vi "tdms读取.vi"() -> ()   [LabVIEW 2018]
panel:
  out "XY图":cluster{"Y":dbl[], "Y":dbl[]}[](graph)
  out "数据":waveform(dbl)[](array[waveform])
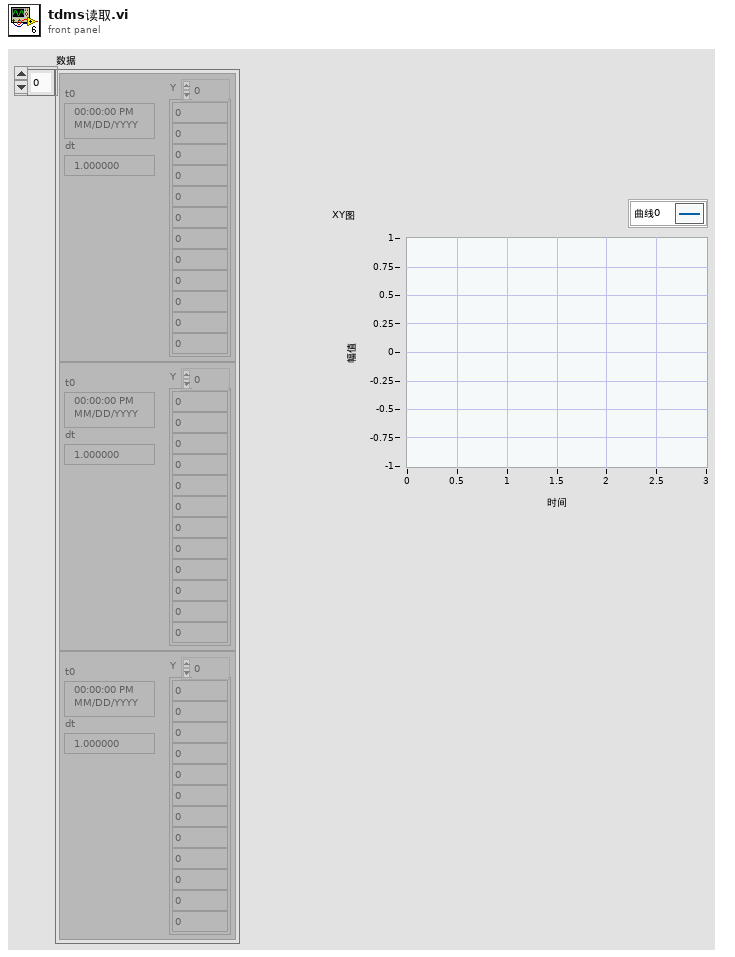
[diagram p1: front panel]
types:
  T1 = enum16{"open", "open or create", "create or replace", "create", "open (read-only)"}
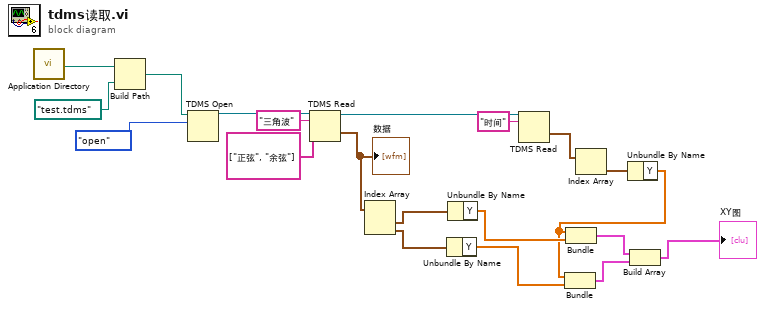
[diagram p0: block diagram]
diagram:
  n1 = call <vilib>:"Application Directory.vi"() -> ("Application Directory"=w19:path)
  n2 = Build Path(base path=w19, name or relative path=path "test.tdms") -> (appended path=w18:path)
  n3 = TDMS Open(10:T1."open" ("操作(0:open)"), 11:w18) -> (3:w16:refnum<k34>)  [unwired: 5 in, 1 out]
  n4 = TDMS Read(0:w16, 5:"三角波" ("组名称输入"), 7:string[] ["正弦", "余弦"] ("通道名称输入")) -> (4:w10:refnum<k34>, 10:w13:waveform(dbl)[])  [unwired: 5 in, 4 out]
  "数据" <- w13
  n5 = Index Array(array=w13) -> (element #1=w12:waveform(dbl), element #2=w11:waveform(dbl))  [unwired: 2 in]
  n6 = Unbundle By Name(w11) -> ("Y"=w4:dbl[])
  n7 = Unbundle By Name(w12) -> ("Y"=w6:dbl[])
  n8 = TDMS Read(0:w10, 5:"时间" ("组名称输入")) -> (10:w8:waveform(dbl)[])  [unwired: 6 in, 5 out]
  n9 = Index Array(array=w8) -> (element=w7:waveform(dbl))  [unwired: 1 in]
  n10 = Unbundle By Name(w7) -> ("Y"=w5:dbl[])
  n11 = Bundle("Y"=w5, "Y"=w4) -> (w3:cluster{"Y":dbl[], "Y":dbl[]})  [unwired: 1 in]
  n12 = Bundle("Y"=w5, "Y"=w6) -> (w2:cluster{"Y":dbl[], "Y":dbl[]})  [unwired: 1 in]
  n13 = Build Array(w2, w3) -> (→"XY图":cluster{"Y":dbl[], "Y":dbl[]}[])
